vi "Remove Percent Codes from String.vi"(11 "String in":string) -> (3 "String out":string)   [LabVIEW 2015, in "NI_AWS_IAM.lvlib"]
uses:
  NI_AWS_IAM.lvlib
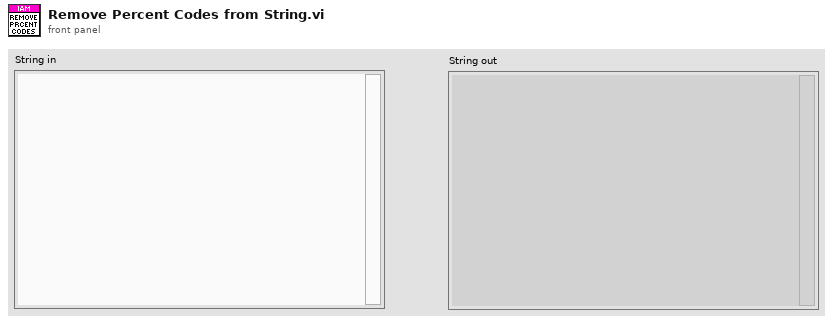
[diagram p1: front panel]
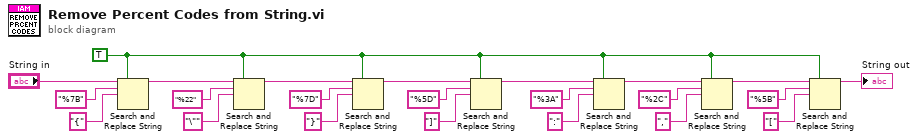
[diagram p0: block diagram]
diagram:
  w1 = TRUE ("replace all? (F)")
  n1 = Search and Replace String(replace all?=w1, input string="String in", search string="%7B", replace string="{" ("search string")) -> (result string=w17:string)  [unwired: 4 in, 3 out]
  n2 = Search and Replace String(replace all?=w1, input string=w17, search string="%22", replace string="\"" ("search string")) -> (result string=w16:string)  [unwired: 4 in, 3 out]
  n3 = Search and Replace String(replace all?=w1, input string=w16, search string="%7D", replace string="}" ("search string")) -> (result string=w15:string)  [unwired: 4 in, 3 out]
  n4 = Search and Replace String(replace all?=w1, input string=w15, search string="%5D", replace string="]" ("search string")) -> (result string=w9:string)  [unwired: 4 in, 3 out]
  n5 = Search and Replace String(replace all?=w1, input string=w9, search string="%3A", replace string=":" ("search string")) -> (result string=w6:string)  [unwired: 4 in, 3 out]
  n6 = Search and Replace String(replace all?=w1, input string=w6, search string="%2C", replace string="," ("search string")) -> (result string=w3:string)  [unwired: 4 in, 3 out]
  n7 = Search and Replace String(replace all?=w1, input string=w3, search string="%5B", replace string="[" ("search string")) -> (result string=→"String out":string)  [unwired: 4 in, 3 out]
